vi "PressureB.vi"() -> ()   [LabVIEW 2015]
uses:
  <vilib>/myRIO/Instrument Drivers/Onboard IO/I2C/typedefs/I2C User Configuration.ctl
  <vilib>/myRIO/Instrument Drivers/Onboard IO/I2C/typedefs/I2C Transfer Rate.ctl
  <vilib>/myRIO/Common/Instrument Driver Framework/myRIO v1.0/UART/vis/myRIO v1.0 Close UART.vi
  <vilib>/Utility/error.llb/Error Cluster From Error Code.vi
  <vilib>/myRIO/Common/Instrument Driver Framework/myRIO v1.0/I2C/vis/myRIO v1.0 Configure I2C.vi
  <vilib>/myRIO/Common/Instrument Driver Framework/myRIO v1.0/I2C/vis/myRIO v1.0 Write I2C.vi
  <vilib>/myRIO/Common/Instrument Driver Framework/myRIO v1.0/I2C/vis/myRIO v1.0 Read I2C.vi
  <vilib>/myRIO/Common/Instrument Driver Framework/Utilities/vis/FPGA Ref Manager.vi
  <vilib>/myRIO/Common/Instrument Driver Framework/myRIO v1.0/myRIO v1.0 Reset FPGA.vi
  <vilib>/myRIO/Common/Instrument Driver Framework/myRIO v1.0/IRQ/vis/myRIO v1.0 IRQ Info FGV.vi
  <vilib>/myRIO/Common/Instrument Driver Framework/myRIO v1.0/IRQ/vis/myRIO v1.0 Timer IRQ Info FGV.vi
  <vilib>/myRIO/Common/Instrument Driver Framework/myRIO v1.0/IRQ/vis/myRIO v1.0 ISR Agent.vi
  <vilib>/myRIO/Instrument Drivers/Onboard IO/I2C/I2C.lvlib
  <vilib>/myRIO/Instrument Drivers/Utilities/Utilities.lvlib
panel:
  out "output cluster":cluster{i16, i16, i16, i16, i16, i16, i16, i16}
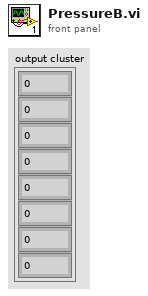
[diagram p1: front panel]
types:
  T1 = typedef "I2C.lvlib/I2C User Configuration.ctl" = cluster{"I2C Transfer Rate":T2}
  T2 = typedef "I2C.lvlib/I2C Transfer Rate.ctl" = enum16{"Standard mode (100 kbps)", "Fast mode (400 kbps)"}
  T3 = typedef "I2C.lvlib/I2C Reference.ctl" = cluster{"myRIO Reference":T4, "I2C Channels Enum":T8, "I2C Configuration":T9}
  T4 = typedef "myRIO Generic Hardware Reference.ctl" = cluster{"myRIO Model":T5, "myRIO Hardware Reference":T6}
  T5 = typedef "Hardware Version Enum.ctl" = enum16{"Unknown", "myRIO-1900", "myRIO-1950", "roboRIO"}
  T6 = typedef "myRIO v1.0 Reference.ctl" = cluster{"Generic FPGA Reference":T7, "Allow multiple opens":bool}
  T7 = typedef "Generic FPGA Reference.ctl" = refnum<k20>
  T8 = typedef "I2C Channels Enum.ctl" = enum16{"Not Connected", "A/I2C", "B/I2C", "I2C/I2C"}
  T9 = typedef "I2C.lvlib/I2C Configuration.ctl" = cluster{"I2C Transfer Rate":T2}
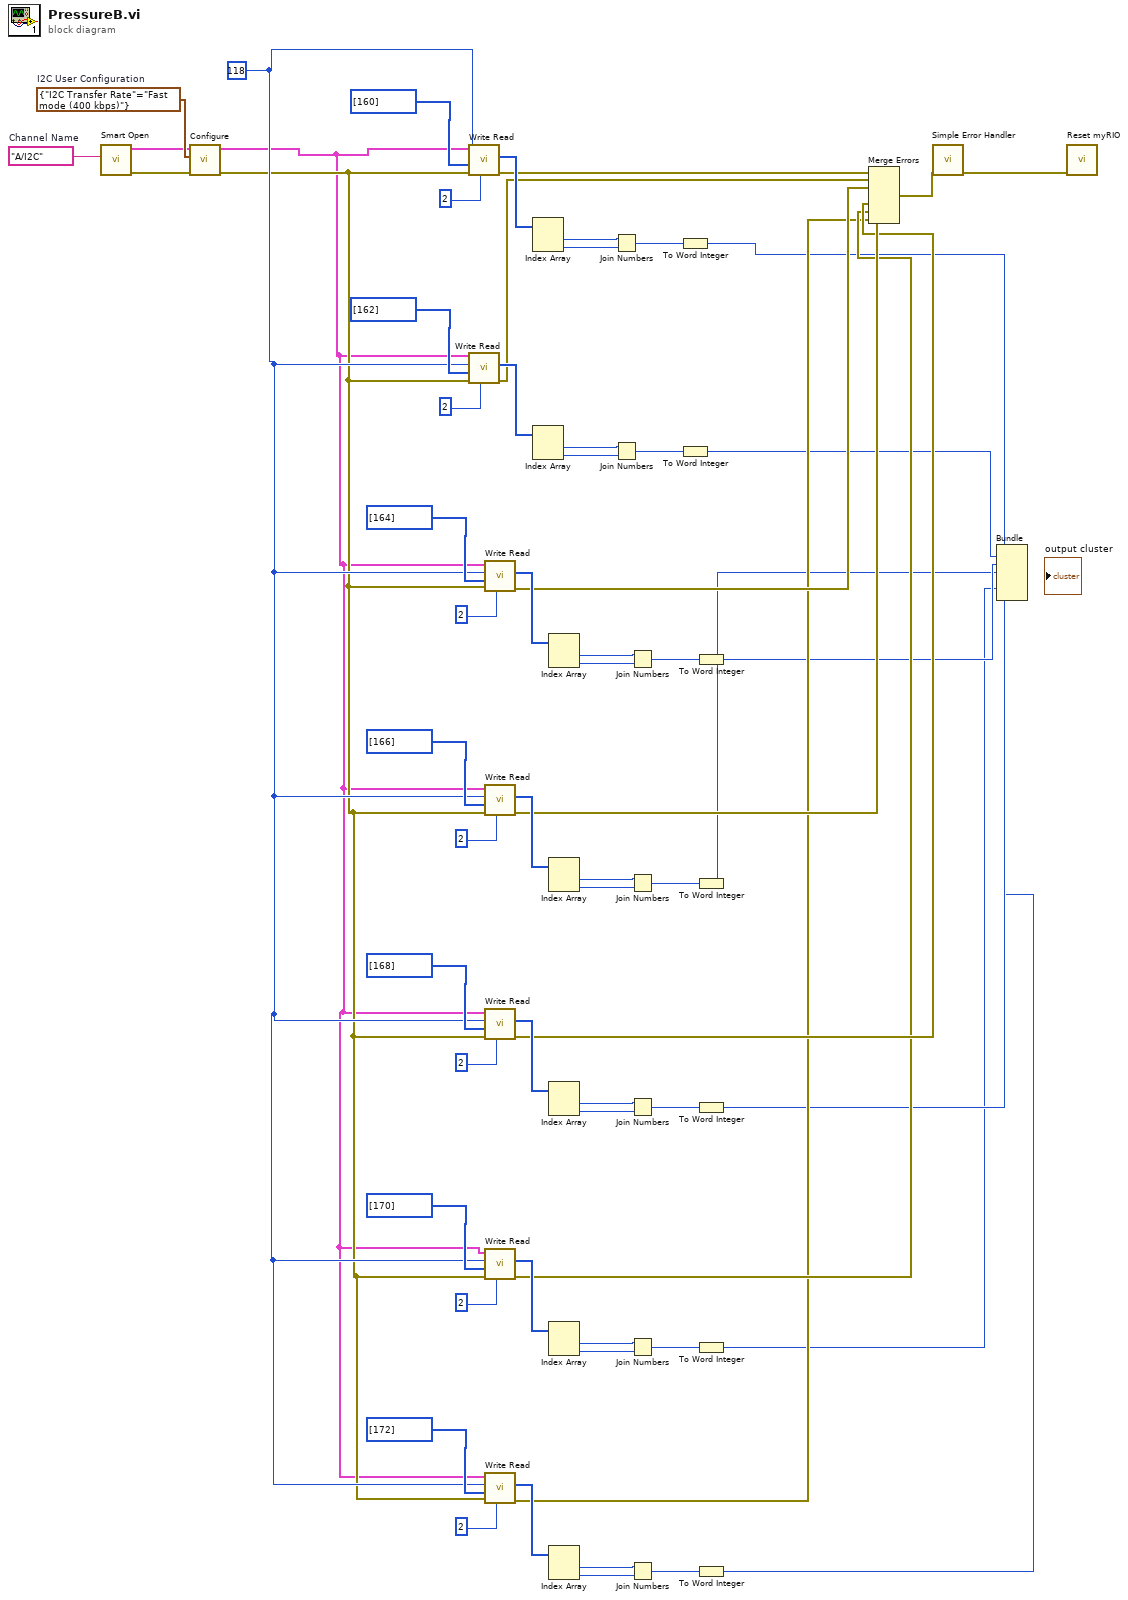
[diagram p0: block diagram]
diagram:
  w18 = u8 118 ("Slave Address (7-bit)")
  w64 = T1 {"I2C Transfer Rate"=enum."Fast mode (400 kbps)"}  # I2C User Configuration
  w65 = tag "A/I2C"  # Channel Name
  n1 = call <vilib>:"Smart Open.vi"("Channel Name"=w65) -> ("error out"=w62:errorcluster, "I2C Ref Out"=w63:T3)  [unwired: 9 in]
  n2 = call <vilib>:"Configure.vi"("error in (no error)"=w62, "I2C User Configuration"=w64, "I2C Ref In"=w63) -> ("error out"=w2:errorcluster, "I2C Ref Out"=w1:T3)  [unwired: 7 in]
  n3 = call <vilib>:"Write Read.vi"("Byte Count"=u32 2, "error in (no error)"=w2, "Bytes to Write"=u8[] [160], "Slave Address (7-bit)"=w18, "I2C Ref In"=w1) -> ("error out"=w17:errorcluster, "Bytes Read"=w56:u8[])  [unwired: 3 in, 1 out]
  n4 = call <vilib>:"Write Read.vi"("Byte Count"=u32 2, "error in (no error)"=w2, "Bytes to Write"=u8[] [162], "Slave Address (7-bit)"=w18, "I2C Ref In"=w1) -> ("error out"=w16:errorcluster, "Bytes Read"=w50:u8[])  [unwired: 3 in, 1 out]
  n5 = call <vilib>:"Write Read.vi"("Byte Count"=u32 2, "error in (no error)"=w2, "Bytes to Write"=u8[] [164], "Slave Address (7-bit)"=w18, "I2C Ref In"=w1) -> ("error out"=w15:errorcluster, "Bytes Read"=w44:u8[])  [unwired: 3 in, 1 out]
  n6 = call <vilib>:"Write Read.vi"("Byte Count"=u32 2, "error in (no error)"=w2, "Bytes to Write"=u8[] [166], "Slave Address (7-bit)"=w18, "I2C Ref In"=w1) -> ("error out"=w14:errorcluster, "Bytes Read"=w38:u8[])  [unwired: 3 in, 1 out]
  n7 = call <vilib>:"Write Read.vi"("Byte Count"=u32 2, "error in (no error)"=w2, "Bytes to Write"=u8[] [168], "Slave Address (7-bit)"=w18, "I2C Ref In"=w1) -> ("error out"=w13:errorcluster, "Bytes Read"=w32:u8[])  [unwired: 3 in, 1 out]
  n8 = call <vilib>:"Write Read.vi"("Byte Count"=u32 2, "error in (no error)"=w2, "Bytes to Write"=u8[] [170], "Slave Address (7-bit)"=w18, "I2C Ref In"=w1) -> ("error out"=w12:errorcluster, "Bytes Read"=w26:u8[])  [unwired: 3 in, 1 out]
  n9 = call <vilib>:"Write Read.vi"("Byte Count"=u32 2, "error in (no error)"=w2, "Bytes to Write"=u8[] [172], "Slave Address (7-bit)"=w18, "I2C Ref In"=w1) -> ("error out"=w11:errorcluster, "Bytes Read"=w20:u8[])  [unwired: 3 in, 1 out]
  n10 = Index Array "Index Array"(array=w56) -> (element #1=w57:u8, element #2=w55:u8)  [unwired: 2 in]
  n11 = Index Array "Index Array"(array=w50) -> (element #1=w51:u8, element #2=w49:u8)  [unwired: 2 in]
  n12 = Index Array "Index Array"(array=w44) -> (element #1=w45:u8, element #2=w43:u8)  [unwired: 2 in]
  n13 = Index Array "Index Array"(array=w38) -> (element #1=w39:u8, element #2=w37:u8)  [unwired: 2 in]
  n14 = Index Array "Index Array"(array=w32) -> (element #1=w33:u8, element #2=w31:u8)  [unwired: 2 in]
  n15 = Index Array "Index Array"(array=w26) -> (element #1=w27:u8, element #2=w25:u8)  [unwired: 2 in]
  n16 = Index Array "Index Array"(array=w20) -> (element #1=w21:u8, element #2=w19:u8)  [unwired: 2 in]
  n17 = Join Numbers(hi=w57, lo=w55) -> ((hi.lo)=w60:u16)
  n18 = Join Numbers(hi=w51, lo=w49) -> ((hi.lo)=w54:u16)
  n19 = Join Numbers(hi=w45, lo=w43) -> ((hi.lo)=w48:u16)
  n20 = Join Numbers(hi=w39, lo=w37) -> ((hi.lo)=w42:u16)
  n21 = Join Numbers(hi=w33, lo=w31) -> ((hi.lo)=w36:u16)
  n22 = Join Numbers(hi=w27, lo=w25) -> ((hi.lo)=w30:u16)
  n23 = Join Numbers(hi=w21, lo=w19) -> ((hi.lo)=w24:u16)
  n24 = To Word Integer(number=w60) -> (16bit integer=w9:i16)
  n25 = To Word Integer(number=w54) -> (16bit integer=w8:i16)
  n26 = To Word Integer(number=w48) -> (16bit integer=w7:i16)
  n27 = To Word Integer(number=w42) -> (16bit integer=w6:i16)
  n28 = To Word Integer(number=w36) -> (16bit integer=w5:i16)
  n29 = To Word Integer(number=w30) -> (16bit integer=w4:i16)
  n30 = To Word Integer(number=w24) -> (16bit integer=w3:i16)
  n31 = Merge Errors(w17, w16, w15, w14, w13, w12, w11) -> (w10:errorcluster)
  n32 = call <vilib>:"Simple Error Handler.vi"("error in (no error)"=w10) -> ("error out"=w61:errorcluster)  [unwired: 4 in, 4 out]
  n33 = Bundle(w9, w8, w7, w6, w5, w4, w3) -> ()  [unwired: 1 in, 1 out]
  n34 = call <vilib>:"Reset myRIO.vi"("error in (no error)"=w61) -> ()  [unwired: 10 in, 1 out]
